vi "core_robust_set_cursor_state.vi"(6 "set/unset (set)":enum16{"set", "unset"}(ring), 8 "error in (no error)":errorcluster, 11 "disable click? (T)":bool=TRUE) -> (0 "error out":errorcluster, 3 "front pannel is closed?":bool)   [LabVIEW 2015]
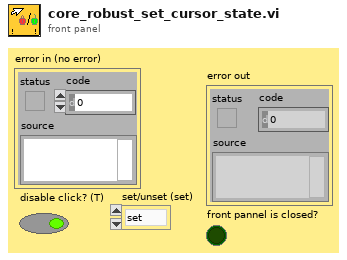
[diagram p1: front panel]
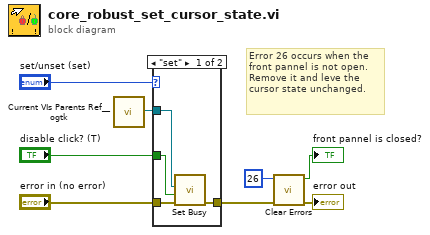
[diagram p0: block diagram]
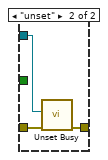
[diagram p2: hidden frame]
diagram:
  # "Error 26 occurs when the front pannel is not open.\nRemove it and leve the cursor state unchanged."
  n1 = call <userlib>:"Current VIs Parents Ref__ogtk.vi"() -> ("Calling VI's Reference"=w7:refnum<vi>)  [unwired: 2 in]
  n2 = case shown="\"set\"" "set/unset (set)" {
    tunnel: "error in (no error)" -> [w12 w14]
    tunnel: w7 -> [w11 w15]
    tunnel: "disable click? (T)" -> [w10 _]
    tunnel: [w9 w13] -> w5
    frame "set" {
      n3 = call <vilib>:"Set Busy.vi"("error in (no error)"=w12, "disable click? (T)"=w10, "VI reference (current VI)"=w11) -> ("error out"=w9:errorcluster)  [unwired: 7 in, 1 out]
    }
    frame "unset" {
      n4 = call <vilib>:"Unset Busy.vi"("error in (no error)"=w14, "VI reference (current VI)"=w15) -> ("error out"=w13:errorcluster)  [unwired: 9 in]
    }
  }
  n5 = call <vilib>:"Clear Errors.vi"("error in (no error)"=w5, "specific error code to clear (0: all)"=26) -> ("error out"=→"error out":errorcluster, "specific error cleared?"=→"front pannel is closed?":bool)  [unwired: 4 in]
